vi "Add Databases Section.vi"(7 "Highlight? (F)":bool, 8 "error in":errorcluster, 11 "Custom device Ref":T1 format="%.0x") -> (0 "error out":errorcluster, 3 "Custom device Ref out":T1 format="%.0x")   [LabVIEW 2020, in "Communication Bus Template Scripting.lvlib"]
uses:
  Communication Bus Template Scripting.lvlib
  <vilib>/NI VeriStand/Custom Device API/Custom Device Item Ref.ctl
  Shared/Constants.vi
  <vilib>/NI VeriStand/Custom Device API/Custom Device API.lvlib
  Shared/Communication Bus Template Shared.lvlib
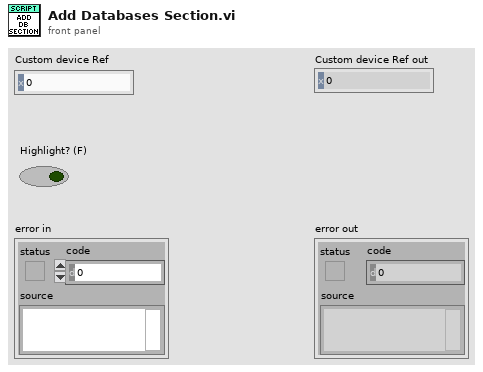
[diagram p1: front panel]
types:
  T1 = typedef "Custom Device API.lvlib/Custom Device Item Ref.ctl" = u64
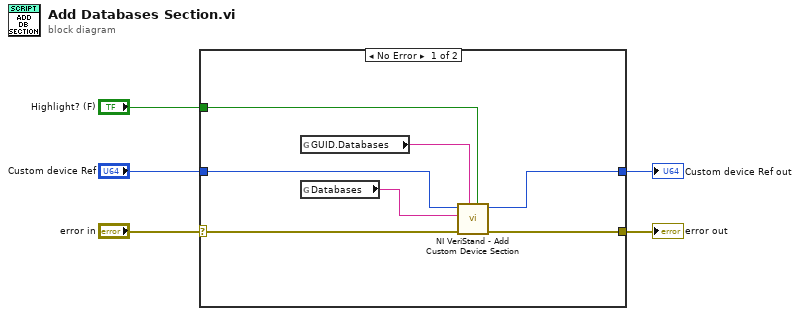
[diagram p0: block diagram]
diagram:
  n1 = case shown="No Error" "error in" {
    selector: "error in" -> [w8 w14]
    tunnel: "Custom device Ref" -> [w11 w13]
    tunnel: [w12 w14] -> w4
    tunnel: "Highlight? (F)" -> [w9 _]
    tunnel: [w6 w13] -> w1
    frame No Error {
      n2 = global read "Constants.vi" "GUID.Databases"() -> (w10:string)
      n3 = global read "Constants.vi" "Databases"() -> (w7:string)
      n4 = call <vilib>:"NI VeriStand - Add Custom Device Section.vi"("Highlight? (F)"=w9, "GUID (Default Section)"=w10, "error in (no error)"=w8, "Section Name"=w7, "Parent Ref in"=w11) -> ("error out"=w12:errorcluster, "Parent Ref out"=w6:T1)  [unwired: 3 in, 2 out]
    }
    frame Error {
    }
  }
  "error out" <- w4
  "Custom device Ref out" <- w1
